vi "Align3DPointSetToPlaneArbitrary.vi"(8 "error in":errorcluster, 10 "Plane Coefficients":T1, 11 "Point Set":T2[](array[typedef])) -> (0 "error out":errorcluster, 3 "Points Aligned to Plane":T2[](array[typedef]))   [LabVIEW 2020, in "ar.lvlib"]
doc: "Align 3D Points to a plane computed based on a Least Mean Squares plane-finding algorithm."
uses:
  ar.lvlib
  Plane Coefficients.ctl
  common/Object Point (Float).ctl
  common/common.lvlib
  Plane Alignment Coefficients.ctl
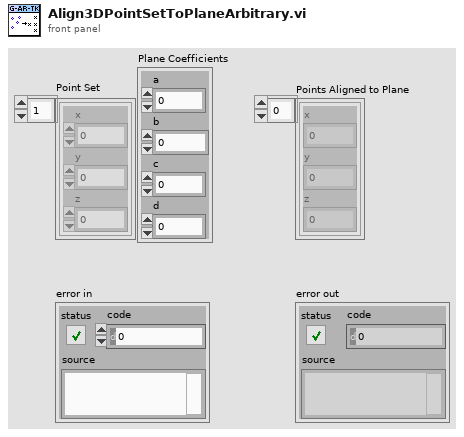
[diagram p1: front panel]
types:
  T1 = typedef "ar.lvlib/Plane Alignment Coefficients.ctl" = cluster{"a":dbl, "b":dbl, "c":dbl, "d":dbl}
  T2 = typedef "common.lvlib/Object Point (Float).ctl" = cluster{"x":dbl, "y":dbl, "z":dbl}
  T3 = typedef "ar.lvlib/Plane Coefficients.ctl" = cluster{"a":dbl, "b":dbl, "c":dbl, "d":dbl}
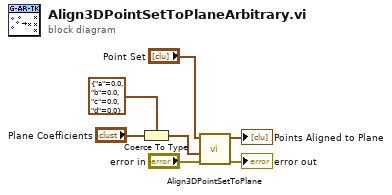
[diagram p0: block diagram]
diagram:
  n1 = Coerce To Type(0:"Plane Coefficients", 1:T3 {"a"=0.0, "b"=0.0, "c"=0.0, "d"=0.0} ("Plane Coeffcients")) -> (2:w3:T3)
  n2 = call "Align3DPointSetToPlane.vi"("error in"="error in", "Plane Coefficients"=w3, "Point Set"="Point Set") -> ("error out"=→"error out":errorcluster, "Points Fitted to Plane"=→"Points Aligned to Plane":T2[])  [unwired: 7 in]
